vi "Place Order.vi"(8 "error in (no error)":errorcluster, 9 "Order To Place":refnum<class "Order.lvclass">, 11 "Agent In":refnum<class "Agent.lvclass">) -> (0 "error out":errorcluster, 3 "Agent Out":refnum<class "Agent.lvclass">)   [LabVIEW 2019, in "Agent.lvclass"]
doc: "Agent (invoker) places order (command) into the queue. The order will not be sent to the stock trader (receiver) until execute order is called."
uses:
  Agent.lvclass
  Order/Order.lvclass
  Agent.lvclass/Agent.ctl
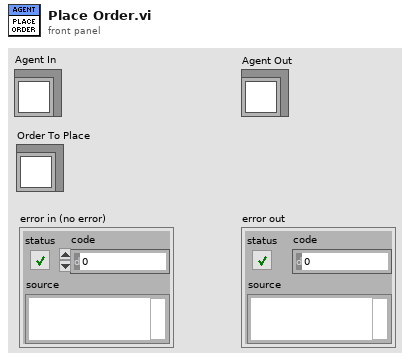
[diagram p1: front panel]
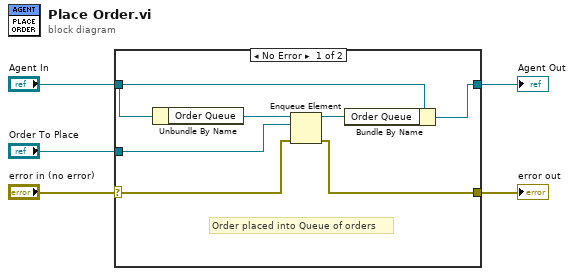
[diagram p0: block diagram]
diagram:
  n1 = case shown="No Error" "error in (no error)" {
    selector: "error in (no error)" -> [w10 w13]
    tunnel: "Order To Place" -> [w11 _]
    tunnel: "Agent In" -> [w9 w14]
    tunnel: [w7 w14] -> w2
    tunnel: [w6 w13] -> w1
    frame No Error {
      # "Order placed into Queue of orders"
      n2 = Unbundle By Name(w9) -> ("Order Queue"=w12:refnum<queue>)
      n3 = Enqueue Element(queue=w12, element=w11, error in (no error)=w10) -> (queue out=w8:refnum<queue>, error out=w6:errorcluster)  [unwired: 1 in, 1 out]
      n4 = Bundle By Name(cluster=w9, "Order Queue"=w8) -> (w7:refnum<class "Agent.lvclass">)
    }
    frame Error {
      # "don't place orders in an error state"
    }
  }
  "Agent Out" <- w2
  "error out" <- w1
